vi "CameraAttributeTest.vi"() -> ()   [LabVIEW 2021]
uses:
  <vilib>/userDefined/High Color/IMAQdx.ctl
  <resource>/objmgr/imaqdx.rc
  <vilib>/vision/driver/NI_Vision_Acquisition_Software.lvlib
panel:
  out "ValueString":string
  out "EnumStrings[] 2":string[](array[string])
  out "EnumStrings[]":string[](array[string])
  in  "Session In":T1
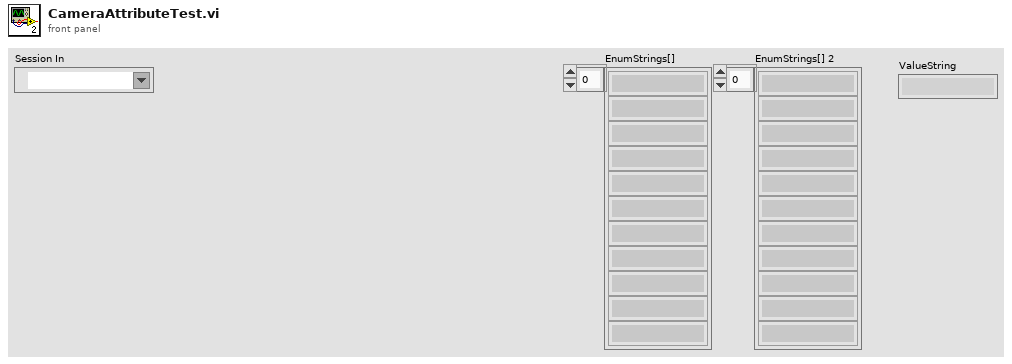
[diagram p1: front panel]
types:
  T1 = typedef "IMAQdx.ctl" = refnum<k21>
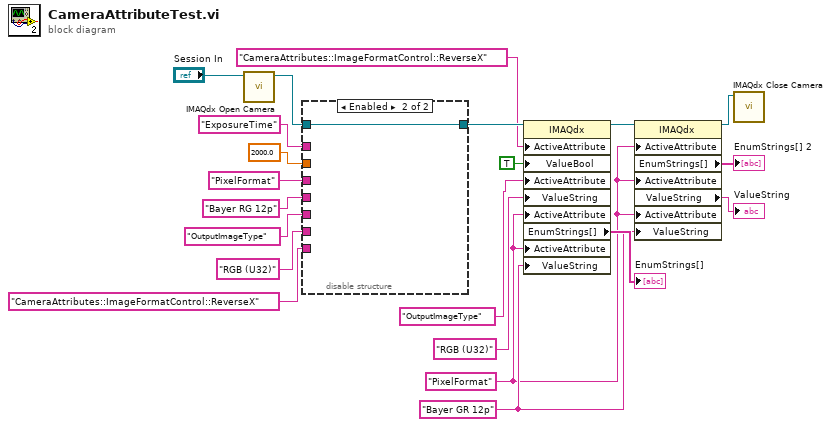
[diagram p0: block diagram]
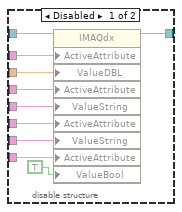
[diagram p2: hidden frame]
diagram:
  w5 = "PixelFormat" ("ActiveAttribute")
  w8 = "Bayer GR 12p" ("ValueString")
  n1 = call <vilib>:"IMAQdx Open Camera.vi"("Session In"="Session In") -> ("Session Out"=w7:T1)  [unwired: 9 in, 1 out]
  n2 = disable-structure shown="Enabled" {
    disable-tunnel: "OutputImageType" ("ActiveAttribute") -> [w31 _]
    disable-tunnel: "RGB (U32)" ("ValueString") -> [w30 _]
    disable-tunnel: "PixelFormat" ("ActiveAttribute") -> [w29 _]
    disable-tunnel: "ExposureTime" ("ActiveAttribute") -> [w28 _]
    disable-tunnel: 2000.0 ("ValueDBL") -> [w27 _]
    disable-tunnel: "CameraAttributes::ImageFormatControl::ReverseX" ("ActiveAttribute") -> [w26 _]
    disable-tunnel: "Bayer RG 12p" ("ValueString") -> [w24 _]
    disable-tunnel: w7 -> [w23 w32]
    disable-tunnel: [w22 w32] -> w6
    frame Disabled {
      n3 = property class="IMAQdx"(reference=w23, "ActiveAttribute"=w28, "ValueDBL"=w27, "ActiveAttribute"=w29, "ValueString"=w24, "ActiveAttribute"=w31, "ValueString"=w30, "ActiveAttribute"=w26, "ValueBool"=TRUE) -> (reference out=w22:T1)  [unwired: 1 in, 1 out]
    }
    frame Enabled {
    }
  }
  n4 = property class="IMAQdx"(reference=w6, "ActiveAttribute"="CameraAttributes::ImageFormatControl::ReverseX", "ValueBool"=TRUE, "ActiveAttribute"="OutputImageType", "ValueString"="RGB (U32)", "ActiveAttribute"=w5, "ActiveAttribute"=w5, "ValueString"=w8) -> (reference out=w12:T1, "EnumStrings[]"=→"EnumStrings[]":string[])  [unwired: 1 in, 1 out]
  n5 = property class="IMAQdx"(reference=w12, "ActiveAttribute"=w5, "ActiveAttribute"=w5, "ActiveAttribute"=w5, "ValueString"=w8) -> (reference out=w11:T1, "EnumStrings[]"=→"EnumStrings[] 2":string[], "ValueString"=→"ValueString":string)  [unwired: 1 in, 1 out]
  n6 = call <vilib>:"IMAQdx Close Camera.vi"("Session In"=w11) -> ()  [unwired: 10 in, 1 out]
